vi "测试数据保存.vi"(7 "文件名称前缀":string, 8 "错误输入（无错误）":errorcluster, 10 "数据":dbl[][](array[numeric]), 11 "start path":path=path "D:/Data") -> (0 "错误输出":errorcluster)   [LabVIEW 2020]
uses:
  <vilib>/Utility/file.llb/Write Delimited Spreadsheet (DBL).vi
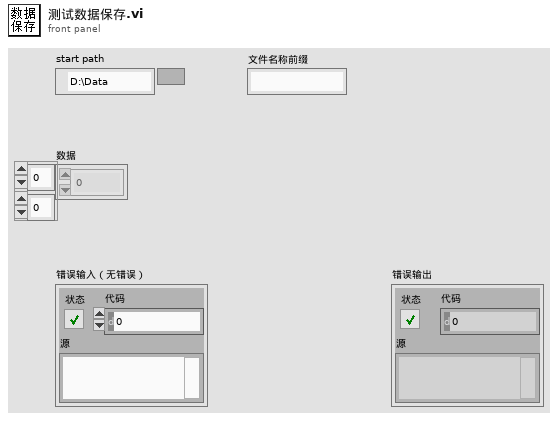
[diagram p1: front panel]
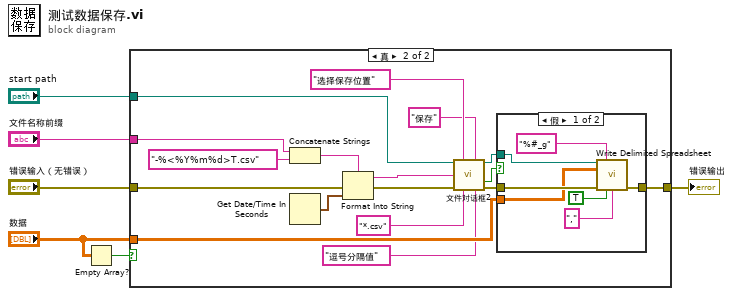
[diagram p0: block diagram]
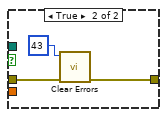
[diagram p3: hidden frame]
diagram:
  n1 = Empty Array?(array="数据") -> (empty?=w5:bool)
  n2 = case shown="真" w5 {
    tunnel: "数据" -> [_ w24]
    tunnel: [w7 w12] -> w3
    tunnel: "错误输入（无错误）" -> [w7 w11]
    tunnel: "文件名称前缀" -> [_ w9]
    tunnel: "start path" -> [_ w8]
    frame False {
    }
    frame True {
      n3 = Concatenate Strings(w9, "-%<%Y%m%d>T.csv" ("格式字符串")) -> (w10:string)
      n4 = Get Date/Time In Seconds() -> (seconds since 1Jan1904=w14:timestamp)
      n5 = Format Into String(format string=w10, error in=w11, w14) -> (resulting string=w16:string, error out=w15:errorcluster)  [unwired: 1 in]
      n6 = call "文件对话框2"("start path"=w8, "prompt"="选择保存位置", "button label"="保存", "default name"=w16, "error in"=w15, "pattern (all files)"="*.csv", "pattern label"="逗号分隔值") -> ("selected path"=w22:path, "cancelled"=w23:bool, "error out"=w20:errorcluster)  [unwired: 5 in, 1 out]
      n7 = case shown="假" w23 {
        tunnel: w20 -> [w31 w34]
        tunnel: [w30 w33] -> w12
        tunnel: w22 -> [w29 _]
        tunnel: w24 -> [w28 _]
        frame False {
          n8 = call-poly <vilib>:"Write Delimited Spreadsheet.vi"("file path (dialog if empty)"=w29, "format (%.3f)"="%#_g", "2D data"=w28, "error in (no error)"=w31, "transpose? (no:F)"=TRUE, "delimiter (\\t)"="," ("delimiter (\\t)")) -> ("error out"=w30:errorcluster)  [unwired: 8 in, 1 out]
        }
        frame True {
          n9 = call <vilib>:"Clear Errors.vi"("error in (no error)"=w34, "specific error code to clear (0: all)"=43) -> ("error out"=w33:errorcluster)  [unwired: 4 in, 1 out]
        }
      }
    }
  }
  "错误输出" <- w3
